vi "WriteConvert Multiple Attributes.vi"(4 "Replace Existing (F)":bool, 5 "Values":variant[](array[variant]), 6 "error in (no error)":errorcluster, 8 "Names":string[](array[string]), 9 "HDF5 Ref":T1) -> (0 "error out":errorcluster, 3 "HDF5 Ref out":T1)   [LabVIEW 2012]
doc: "Takes an array of names and a corresponding array of values and writes them as attributes on the HDF5 object given by HDF5 Ref. If Replace Existing is false and an attribute with the same name already exists, an error will occur."
uses:
  <vilib>/addons/_hdf5/library.llb/HDF5 Ref.ctl
  <vilib>/addons/_hdf5/openg.llb/Type Descriptor Enumeration__ogtk.ctl
panel:
  # "Copyright (C) 2005-2006 by Jason D. Sommerville                 \n\nThis program is free software; you can redistribute it and/or modify  it under the terms of the Common Public License Version 1.0 as  published by the Open Source Initiative.                          \n\nThis program is distributed in the hope that it will be useful, but WITHOUT ANY WARRANTY; without even the implied warranty of  MERCHANTABILITY or FITNESS FOR A PARTICULAR PURPOSE.  See the Common Public License for more details. \n\nYou should have received a copy of the Common Public License along with this program; if not, visit the OSI website at http://www.opensource.org/"
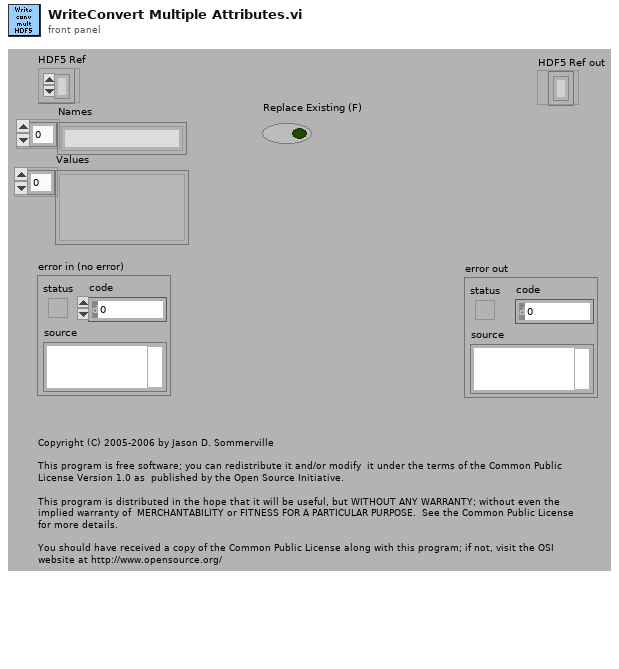
[diagram p1: front panel]
types:
  T1 = typedef "HDF5 Ref.ctl" = refnum<k1>
  T2 = typedef "Type Descriptor Enumeration__ogtk.ctl" = enum8{"<Null>", "I8", "I16", "I32", "I64", "U8", "U16", "U32", "U64", "SGL", "DBL", "EXT", "CSG", "CDB", "CXT", "0x0F", "0x10", "0x11", "0x12", "0x13", "0x14", "Enum U8", "Enum U16", "Enum U32", "Enum U64", "SGL PQ", "DBL PQ", "EXT PQ", "CSG PQ", "CDB PQ", "CXT PQ", "0x1F", "0x20", "Boolean", "0x22", "0x23", "0x24", "0x25", "0x26", "0x27", "0x28", "0x29", "0x2A", "0x2B", "0x2C", "0x2D", "0x2E", "0x2F", "String", "0x31", "Path", "Pict", "0x34", "0x35", "0x36", "DAQ", "0x38", "0x39", "0x3A", "0x3B", "0x3C", "0x3D", "0x3E", "0x3F", "Array", "0x41", "0x42", "0x43", "0x44", "0x45", "0x46", "0x47", "0x48", "0x49", "0x4A", "0x4B", "0x4C", "0x4D", "0x4E", "0x4F", "Cluster", "0x51", "0x52", "Variant", "Waveform", "0x55", "0x56", "0x57", "0x58", "0x59", "0x5A", "0x5B", "0x5C", "0x5D", "0x5E", "0x5F", "0x60", "0x61", "0x62", "0x63", "0x64", "0x65", "0x66", "0x67", "0x68", "0x69", "0x6A", "0x6B", "0x6C", "0x6D", "0x6E", "0x6F", "Refnum"}
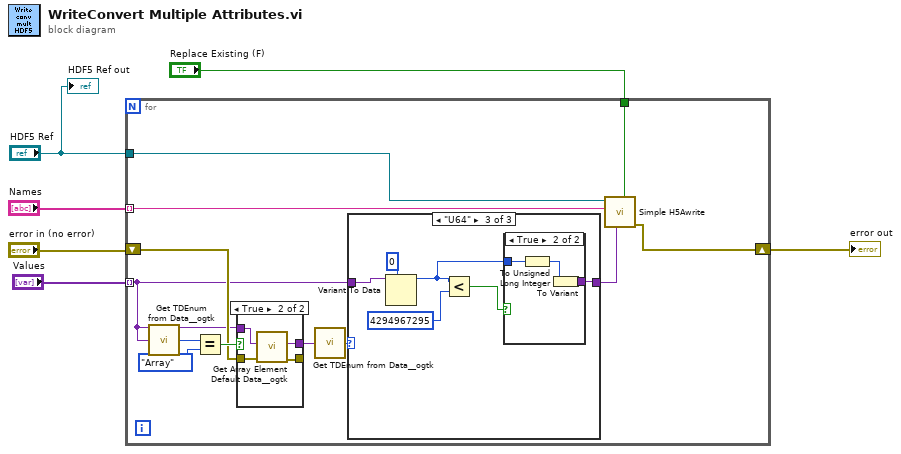
[diagram p0: block diagram]
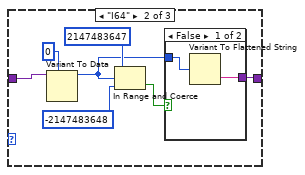
[diagram p3: hidden frame]
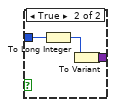
[diagram p4: hidden frame]
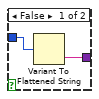
[diagram p5: hidden frame]
diagram:
  n1 = for {
    tunnel: "HDF5 Ref" -> [w17]
    tunnel: "Values" -> [w8] mode=indexing
    shift-right: [w18] -> w3
    shift-left: "error in (no error)" -> [w11]
    tunnel: "Names" -> [w16] mode=indexing
    tunnel: "Replace Existing (F)" -> [w15]
    n2 = call <vilib>:"Get TDEnum from Data__ogtk.vi"("Data"=w8) -> ("Type Descriptor Enumeration"=w14:T2)  [unwired: 4 in]
    n3 = Equal?(x=w14, y=Type_Descriptor_Enumeration__ogtk."Array") -> (x = y?=w12:bool)
    n4 = case shown="True" w12 {
      tunnel: [w43 w45] -> w10
      tunnel: [w44 w47] -> _
      tunnel: w11 -> [w44 w48]
      tunnel: w8 -> [w43 w46]
      frame False {
      }
      frame True {
        n5 = call <vilib>:"Get Array Element Default Data__ogtk.vi"("error in (no error)"=w48, "Array"=w46) -> ("error out"=w47:errorcluster, "Array Element Default Data"=w45:variant)  [unwired: 8 in]
      }
    }
    n6 = call <vilib>:"Get TDEnum from Data__ogtk.vi"("Data"=w10) -> ("Type Descriptor Enumeration"=w9:T2)  [unwired: 4 in]
    n7 = case shown="\"U64\"" w9 {
      tunnel: w8 -> [w19 w26 w37]
      tunnel: [w19 w20 w35] -> w7
      frame "<Null>", Default {
      }
      frame "I64" {
        n8 = Variant To Data(type=i64 0, Variant=w26) -> (data=w21:i64)  [unwired: 1 in, 1 out]
        n9 = In Range and Coerce(upper limit=2147483647, x=w21, lower limit=-2147483648) -> (In Range?=w22:bool)  [unwired: 1 out]
        n10 = case shown="False" w22 {
          tunnel: w21 -> [w28 w31]
          tunnel: [w27 w29] -> w20
          frame False {
            n11 = Variant To Flattened String(Variant=w28) -> (data string=w27:string)  [unwired: 1 out]
          }
          frame True {
            n12 = To Long Integer(number=w31) -> (32bit integer=w30:i32)
            n13 = To Variant(anything=w30) -> (Variant=w29:variant)
          }
        }
      }
      frame "U64" {
        n14 = Variant To Data(type=u64 0, Variant=w37) -> (data=w34:u64)  [unwired: 1 in, 1 out]
        n15 = Less?(x=w34, y=u32 4294967295) -> (x < y?=w32:bool)
        n16 = case shown="True" w32 {
          tunnel: w34 -> [w39 w42]
          tunnel: [w38 w40] -> w35
          frame False {
            n17 = Variant To Flattened String(Variant=w39) -> (data string=w38:string)  [unwired: 1 out]
          }
          frame True {
            n18 = To Unsigned Long Integer(number=w42) -> (unsigned 32bit integer=w41:u32)
            n19 = To Variant(anything=w41) -> (Variant=w40:variant)
          }
        }
      }
    }
    n20 = call <vilib>:"Simple H5Awrite.vi"("Replace Existing (F)"=w15, "Value"=w7, "Name"=w16, "HDF5 Ref"=w17) -> ("error out"=w18:errorcluster)  [unwired: 4 in, 1 out]
  }
  "error out" <- w3
  "HDF5 Ref out" <- "HDF5 Ref"
